vi "Update_FM.vi"(8 "error in (no error)":errorcluster {"code" format="%.0x"}, 9 "channel name (\"1\")":string="1", 10 "FM":T2={"ON/OFF"=FALSE, "source (0: Internal)"=0, "peak deviation (1000000)"=1000000.0, "modulation frequency (10000)"=10000.0, "waveform (1: Sine)"=1} {"waveform (1: Sine)" items=["Sine"=1, "Square"=2, "Pulse"=1002, "Ramp"=1001, "Noise"=1003, "DC"=6, "Sin(x)/x"=1004, "Gaussian"=1005, "Lorentz"=1006, "Exponential Rise"=1007, "Exponential Decay"=1008, "Haversine"=1009]; "source (0: Internal)" items=["Internal", "External"]}, 11 "resource name":refnum<k15>) -> (0 "error out":errorcluster, 2 "output cluster":T1, 3 "instrument handle out":refnum<k15>)   [LabVIEW 2015, in "MyToolsFunction.lvlib"]
uses:
  ICcamera/MyToolsFunction.lvlib
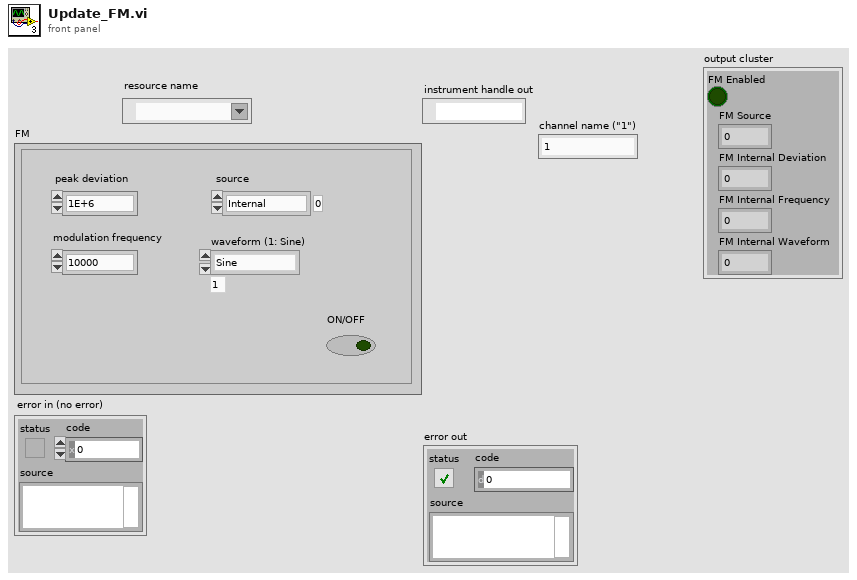
[diagram p1: front panel]
types:
  T1 = cluster{"FM Enabled":bool, "FM Source":i32, "FM Internal Deviation":dbl, "FM Internal Frequency":dbl, "FM Internal Waveform":i32}
  T2 = cluster{"ON/OFF":bool, "source (0: Internal)":i32, "peak deviation (1000000)":dbl, "modulation frequency (10000)":dbl, "waveform (1: Sine)":i32}
  T3 = cluster{"FM Enabled":bool, "FM Source":i32, "FM Deviation By Channel":dbl, "FM Internal Frequency By Channel":dbl, "FM Internal Waveform By Channel":i32}
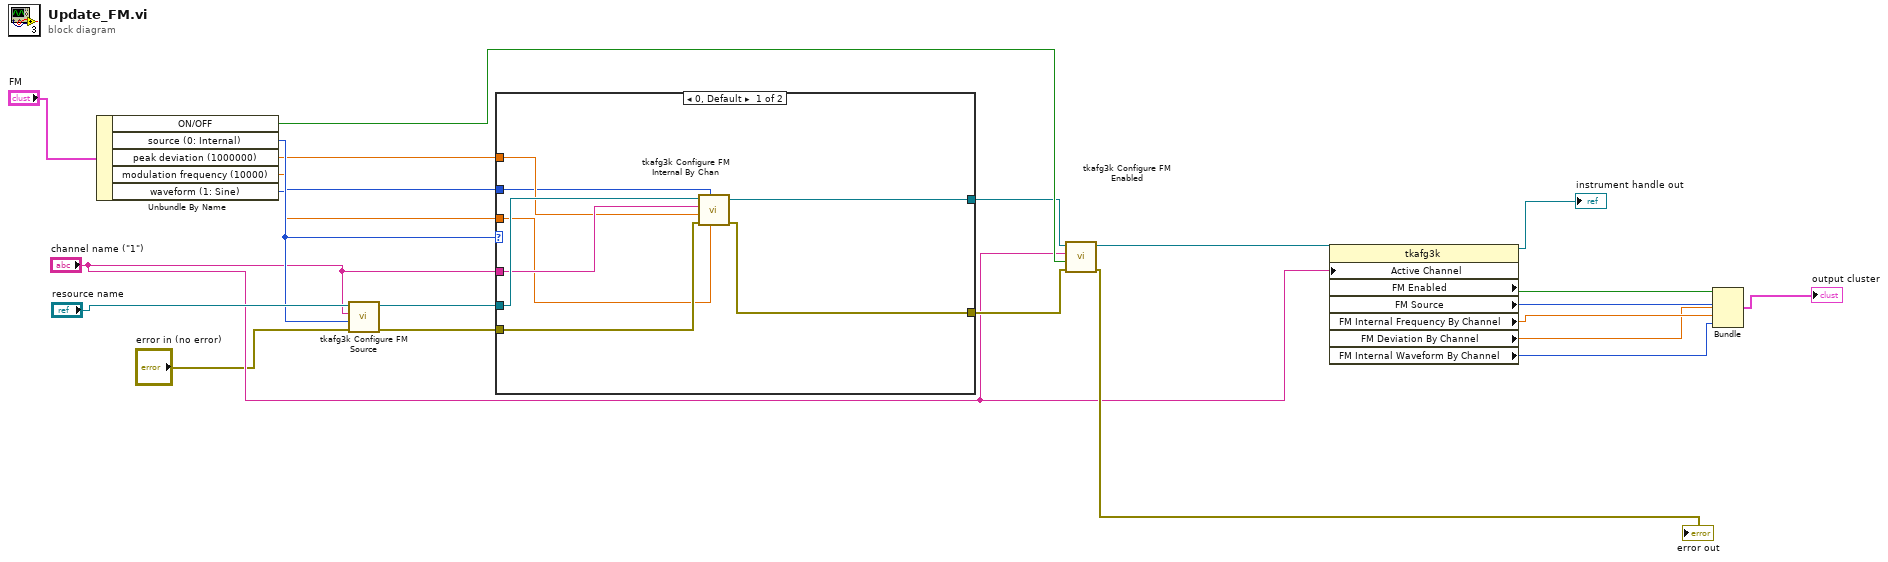
[diagram p0: block diagram]
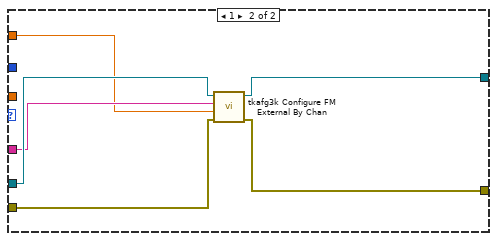
[diagram p2: hidden frame]
diagram:
  n1 = Unbundle By Name("FM") -> ("ON/OFF"=w14:bool, "source (0: Internal)"=w21:i32, "peak deviation (1000000)"=w18:dbl, "modulation frequency (10000)"=w17:dbl, "waveform (1: Sine)"=w12:i32)
  n2 = call <instrlib>:"tkafg3k Configure FM Source.vi"("error in (no error)"="error in (no error)", "source (0: Internal)"=w21, "channel name (\"1\")"="channel name (\"1\")", "instrument handle"="resource name") -> ("error out"=w19:errorcluster, "instrument handle out"=w20:refnum<k15>)  [unwired: 6 in]
  n3 = case shown="0, Default" w21 {
    tunnel: w20 -> [w30 w36]
    tunnel: [w29 w35] -> w11
    tunnel: w19 -> [w28 w33]
    tunnel: [w27 w34] -> w16
    tunnel: "channel name (\"1\")" -> [w26 w32]
    tunnel: w18 -> [w25 w31]
    tunnel: w17 -> [w24 _]
    tunnel: w12 -> [w23 _]
    frame 0, Default {
      n4 = call <instrlib>:"tkafg3k Configure FM Internal By Chan.vi"("Modulation Frequency (10000)"=w24, "Modulation Waveform (1: Sine)"=w23, "error in (no error)"=w28, "Peak Deviation (1000000)"=w25, "Channel Name (\"1\")"=w26, "instrument handle"=w30) -> ("error out"=w27:errorcluster, "instrument handle out"=w29:refnum<k15>)  [unwired: 4 in]
    }
    frame 1 {
      n5 = call <instrlib>:"tkafg3k Configure FM External By Chan.vi"("error in (no error)"=w33, "Peak Deviation (1000000)"=w31, "Channel Name (\"1\")"=w32, "instrument handle"=w36) -> ("error out"=w34:errorcluster, "instrument handle out"=w35:refnum<k15>)  [unwired: 6 in]
    }
  }
  n6 = call <instrlib>:"tkafg3k Configure FM Enabled.vi"("error in (no error)"=w16, "FM enabled (True)"=w14, "channel name (\"1\")"="channel name (\"1\")", "instrument handle"=w11) -> ("error out"=→"error out":errorcluster, "instrument handle out"=w4:refnum<k15>)  [unwired: 6 in]
  n7 = property class="tkafg3k"(reference=w4, "Active Channel"="channel name (\"1\")") -> (reference out=→"instrument handle out":refnum<k15>, "FM Enabled"=w8:bool, "FM Source"=w7:i32, "FM Internal Frequency By Channel"=w6:dbl, "FM Deviation By Channel"=w3:dbl, "FM Internal Waveform By Channel"=w5:i32)  [unwired: 1 in, 1 out]
  n8 = Bundle("FM Enabled"=w8, "FM Source"=w7, "FM Deviation By Channel"=w3, "FM Internal Frequency By Channel"=w6, "FM Internal Waveform By Channel"=w5) -> (→"output cluster":T3)  [unwired: 1 in]
